vi "Update Axis.vi"(8 "error in (no error)":errorcluster, 10 "Axis":T1={"Enabled"=0, "ArrowStyle"=1, "LineWidth"=2, "IsMarginVisible"=FALSE, "IsMarksNextToAxis"=FALSE, "IsReversed"=FALSE, "IsStartedFromZero"=FALSE, "Title"=""} {"ArrowStyle" items=["None", "Triangle", "SharpTriangle", "Lines"]; "Enabled" items=["None", "Triangle", "SharpTriangle", "Lines"]}, 11 ".NET Refnum in":refnum<k24>) -> (0 "error in":errorcluster, 3 ".NET Refnum out":refnum<k24>)   [LabVIEW 2014, in "XMSChart.xctl"]
uses:
  XMSChart.xctl
  System.Windows.Forms.DataVisualization
  Controls/Axis.ctl
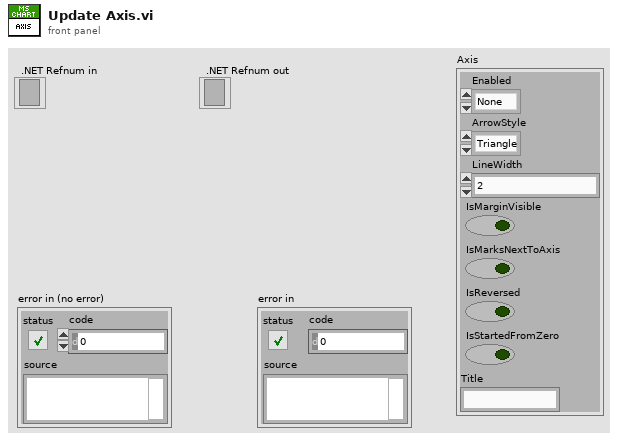
[diagram p1: front panel]
types:
  T1 = typedef "XMSChart.xctl/Axis.ctl" = cluster{"Enabled":i32, "ArrowStyle":i32, "LineWidth":i32, "IsMarginVisible":bool, "IsMarksNextToAxis":bool, "IsReversed":bool, "IsStartedFromZero":bool, "Title":string}
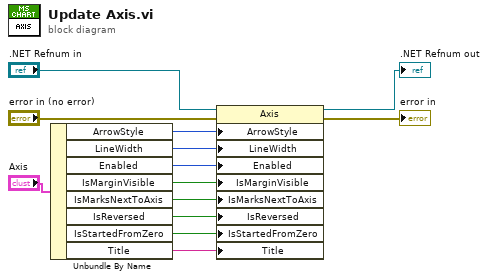
[diagram p0: block diagram]
diagram:
  n1 = Unbundle By Name("Axis") -> ("ArrowStyle"=w11:i32, "LineWidth"=w12:i32, "Enabled"=w6:i32, "IsMarginVisible"=w5:bool, "IsMarksNextToAxis"=w4:bool, "IsReversed"=w3:bool, "IsStartedFromZero"=w2:bool, "Title"=w1:string)
  n2 = property on="Property Node" class="Axis"(reference=".NET Refnum in", error in="error in (no error)", "ArrowStyle"=w11, "LineWidth"=w12, "Enabled"=w6, "IsMarginVisible"=w5, "IsMarksNextToAxis"=w4, "IsReversed"=w3, "IsStartedFromZero"=w2, "Title"=w1) -> (reference out=→".NET Refnum out":refnum<k24>, error out=→"error in":errorcluster)
